vi "SVFA Power Spectrum Subset with Variable Resolution (1 Ch).vi"(0 "scaled signal [EU]":waveform(dbl)={"t0"=timestamp(0 s since 1904-01-01), "dt"=1e-05, "Y"=[]}, 2 "window":T2=1 items=["None"=0, "Hanning"=1, "Hamming"=2, "Blackman-Harris"=3, "Exact Blackman"=4, "Blackman"=5, "Flat Top"=6, "4 Term B-Harris "=7, "7 Term B-Harris"=8, "Low Sidelobe"=9, "Force"=64, "Exponential"=65, "Blackman Nuttall"=11, "Triangle"=30, "Bartlett-Hanning"=31, "Bohman"=32, "Parzen"=33, "Welch"=34, "Kaiser"=60, "Dolph-Chebyshev"=61, "Gaussian"=62], 3 "band specifications [Hz]":T1(array[cluster])=[{"start"=0.0, "stop"=500.0, "resolution"=3.6}, {"start"=500.0, "stop"=1600.0, "resolution"=6.25}, {"start"=1600.0, "stop"=3200.0, "resolution"=12.5}, {"start"=3200.0, "stop"=6400.0, "resolution"=25.0}, {"start"=6400.0, "stop"=12800.0, "resolution"=50.0}, {"start"=12800.0, "stop"=20000.0, "resolution"=100.0}], 4 "dB On (T)":bool=TRUE, 5 "error in (no error)":errorcluster) -> (14 "power spectrum [dB EU]":cluster{"frequencies":dbl[], "magnitudes":dbl[]} {"frequencies" format="%.2f"; "magnitudes" format="%.2p"}, 19 "error out":errorcluster)   [LabVIEW 2017]
uses:
  <vilib>/addons/_NISVFA/_Shared subVIs/Controls/svc_Window.ctl
  <vilib>/addons/_NISVFA/_Shared subVIs/Common/svc_Get Array Subset (Index).vi
  <vilib>/addons/_NISVFA/_Shared subVIs/Common/svc_Coerce Index and Length.vi
  <vilib>/addons/_NISVFA/_Shared subVIs/Common/svc_Conditional Merge Error.vi
  <vilib>/addons/_NISVFA/_Subset FFT/SVFA Power Spectrum Subset (1 Ch).vi
  <vilib>/measure/macond.llb/IIR Filter for 1 Chan.vi
  <vilib>/measure/NI_MAPro.lvlib
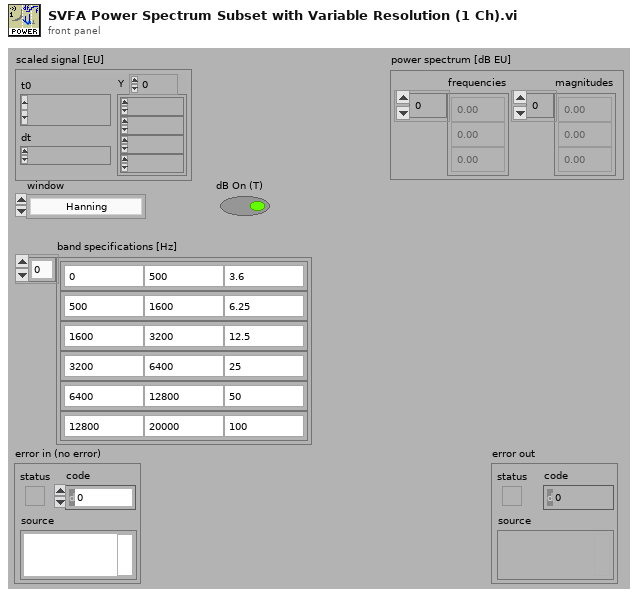
[diagram p1: front panel]
types:
  T1 = cluster{"start":dbl, "stop":dbl, "resolution":dbl}[]
  T2 = typedef "svc_Window.ctl" = u32
  T3 = cluster{"Topology":enum16{"Off", "Butterworth", "Chebyshev", "Inverse Chebyshev", "Elliptic", "Bessel"}, "Type":enum16{"Lowpass", "Highpass", "Bandpass", "Bandstop"}, "Order":i32, "Lower Fc":dbl, "Upper Fc":dbl, "PB Ripple":dbl, "SB Attenuation":dbl}
  T4 = cluster{"averaging mode":enum16{"No averaging", "Vector averaging", "RMS averaging", "Peak hold"}, "weighting mode":enum16{"Linear", "Exponential"}, "number of averages":u32, "linear mode":enum16{"One shot", "Auto restart"}}
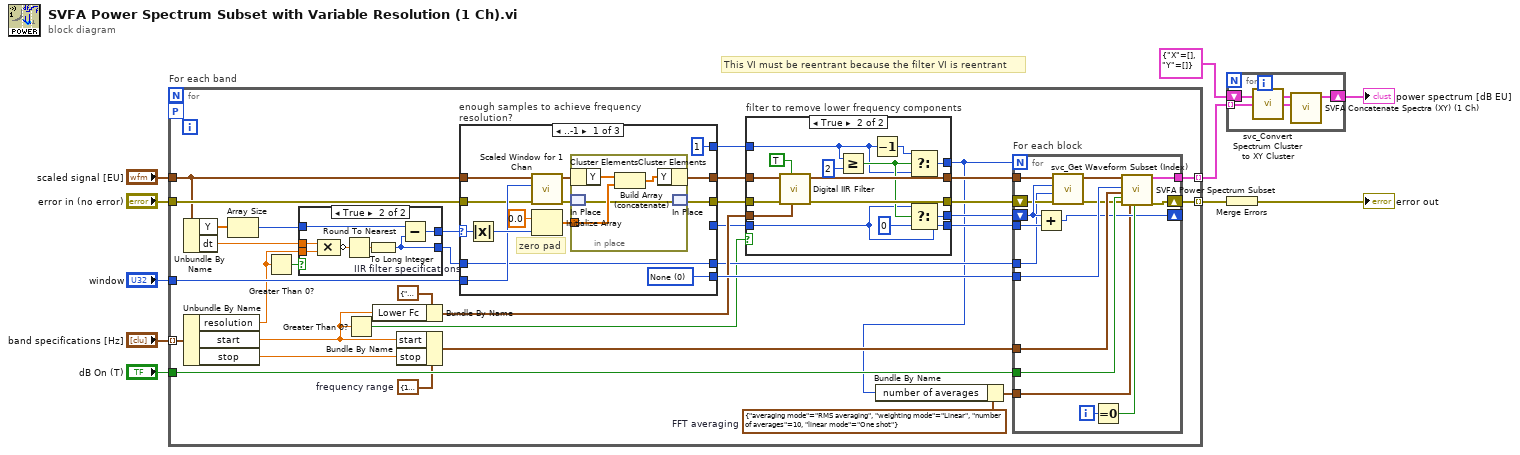
[diagram p0: block diagram]
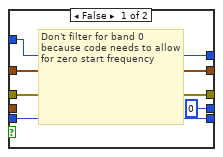
[diagram p2: hidden frame]
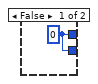
[diagram p3: hidden frame]
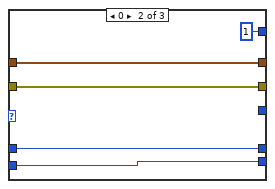
[diagram p4: hidden frame]
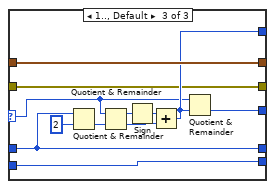
[diagram p5: hidden frame]
diagram:
  # "This VI must be reentrant because the filter VI is reentrant"
  n1 = for "For each band" {
    tunnel: "window" -> [w44]
    tunnel: "dB On (T)" -> [w39]
    tunnel: "band specifications [Hz]" -> [w25] mode=indexing
    tunnel: "scaled signal [EU]" -> [w14]
    tunnel: "error in (no error)" -> [w17]
    tunnel: [w38] -> w6 mode=indexing
    workers-P: _ -> [_]
    tunnel: [w15] -> w3 mode=indexing
    w22 = cluster{"start":dbl, "stop":dbl} {"start"=1000.0, "stop"=2000.0}  # frequency range
    w34 = T3 {"Topology"=enum."Chebyshev", "Type"=enum."Highpass", "Order"=6, "Lower Fc"=100.0, "Upper Fc"=200.0, "PB Ripple"=0.02, "SB Attenuation"=60.0}  # IIR filter specifications
    w36 = T4 {"averaging mode"=enum."RMS averaging", "weighting mode"=enum."Linear", "number of averages"=10, "linear mode"=enum."One shot"}  # FFT averaging
    n2 = Unbundle By Name(w14) -> ("Y"=w12:dbl[], "dt"=w11:dbl)
    n3 = Unbundle By Name(w25) -> ("resolution"=w24:dbl, "start"=w18:dbl, "stop"=w23:dbl)
    n4 = Array Size(array=w12) -> (size(s)=w13:i32)
    n5 = Greater Than 0?(x=w24) -> (x > 0?=w42:bool)
    n6 = case shown="True" w42 {
      tunnel: w11 -> [_ w87]
      tunnel: w24 -> [_ w86]
      tunnel: w13 -> [_ w85]
      tunnel: [w80 w82] -> w43
      tunnel: [w80 w81] -> w37
      frame False {
        w80 = 0
      }
      frame True {
        n7 = Compound Arithmetic op=MULTIPLY(w87, w86) -> (invert w84:dbl)
        n8 = Round To Nearest(number=w84) -> (nearest integer value=w83:dbl)
        n9 = To Long Integer(number=w83) -> (32bit integer=w81:i32)
        n10 = Subtract(x=w85, y=w81) -> (x-y=w82:i32)
      }
    }
    n11 = Greater Than 0?(x=w18) -> (x > 0?=w19:bool)
    n12 = Bundle By Name(cluster=w34, "Lower Fc"=w18) -> (w31:T3)
    n13 = Bundle By Name(cluster=w22, "start"=w18, "stop"=w23) -> (w40:cluster{"start":dbl, "stop":dbl})
    n14 = case "enough samples to achieve frequency resolution?" shown="..-1" w43 {
      selector: w43 -> [w101 _ w111]
      tunnel: w44 -> [w92 w109 w121]
      tunnel: w14 -> [w94 w110 w122]
      tunnel: [w98 w110 w122] -> w33
      tunnel: w37 -> [w91 w107 w113]
      tunnel: [w96 w109 w121] -> w41
      tunnel: [1 1 w115] -> w29
      tunnel: [_ _ w114] -> w28
      tunnel: [w91 w107 w113] -> w21
      tunnel: w17 -> [w90 w106 w112]
      tunnel: [w88 w106 w112] -> w16
      frame ..-1 {
        w96 = T2 0 items=["None"=0, "Hanning"=1, "Hamming"=2, "Blackman-Harris"=3, "Exact Blackman"=4, "Blackman"=5, "Flat Top"=6, "4 Term B-Harris "=7, "7 Term B-Harris"=8, "Low Sidelobe"=9, "Blackman Nuttall"=11, "Triangle"=30, "Bartlett-Hanning"=31, "Bohman"=32, "Parzen"=33, "Welch"=34, "Kaiser"=60, "Dolph-Chebyshev"=61, "Gaussian"=62] ("window")
        # "zero pad"
        n15 = Absolute Value(x=w101) -> (abs(x)=w97:i32)
        n16 = call <vilib>:"Scaled Window for 1 Chan.vi"("error in (no error)"=w90, "window"=w92, "signal in"=w94) -> ("error out"=w89:errorcluster, "signal out"=w93:waveform(dbl))  [unwired: 6 in, 1 out]
        n17 = Initialize Array(0.0 ("element"), w97) -> (w99:dbl[])
        n18 = in-place {
          in-place-border: w99 -> [w104]
          n19 = in-place-cluster #1(w93) -> ("Y"=w105:dbl[])
          n20 = in-place-match #2(w89) -> (w102:errorcluster)
          n21 = Build Array (concatenate)(w105, w104) -> (w103:dbl[])
          n22 = in-place-cluster #1("Y"=w103) -> (w98:waveform(dbl))
          n23 = in-place-match #2(w102) -> (w88:errorcluster)
        }
      }
      frame 0 {
      }
      frame 1.., Default {
        n24 = Quotient & Remainder(x=w113, y=2) -> (floor(x/y)=w119:i32)  [unwired: 1 out]
        n25 = Quotient & Remainder(x=w111, y=w119) -> (x-y*floor(x/y)=w118:i32, floor(x/y)=w116:i32)
        n26 = Sign(1:w118) -> (0:w117:i32)
        n27 = Add(x=w117, y=w116) -> (x+y=w115:i32)
        n28 = Quotient & Remainder(x=w111, y=w115) -> (floor(x/y)=w114:i32)  [unwired: 1 out]
      }
    }
    n29 = case "filter to remove lower frequency components" shown="True" w19 {
      tunnel: w33 -> [w48 w63]
      tunnel: w16 -> [w47 w62]
      tunnel: [w47 w61] -> w32
      tunnel: w31 -> [_ w60]
      tunnel: [w48 w59] -> w30
      tunnel: w29 -> [w49 w52]
      tunnel: [w49 w53] -> w20
      tunnel: w28 -> [w46 w51]
      tunnel: [w46 w51] -> w27
      tunnel: [0 ("f") w54] -> w26
      frame False {
        # "Don't filter for band 0 because code needs to allow for zero start frequency"
      }
      frame True {
        n30 = call-poly <vilib>:"Digital IIR Filter.vi"("IIR filter specifications"=w60, "reset filter"=TRUE, "error in (no error)"=w62, "signal in"=w63) -> ("error out"=w61:errorcluster, "signal out"=w59:waveform(dbl))  [unwired: 5 in, 1 out]
        n31 = Greater Or Equal?(x=w52, y=2) -> (x >= y?=w56:bool)
        n32 = Decrement(x=w52) -> (x-1=w57:i32)
        n33 = Select(t=w57, s=w56, f=w52) -> (s? t:f=w53:i32)
        n34 = Select(t=w51, s=w56, f=0) -> (s? t:f=w54:i32)
      }
    }
    n35 = Bundle By Name(cluster=w36, "number of averages"=w20) -> (w35:T4)
    n36 = for "For each block" {
      N: w20 -> [_]
      tunnel: w41 -> [w79]
      tunnel: [w78] -> w15
      tunnel: w40 -> [w75]
      tunnel: w39 -> [w74]
      shift-right: [w65] -> w38
      shift-left: w32 -> [w67]
      shift-right: [w70] -> _
      shift-left: w26 -> [w71]
      tunnel: w27 -> [w72]
      tunnel: w35 -> [w69]
      tunnel: w30 -> [w68]
      tunnel: w21 -> [w64]
      i -> [w77]
      n37 = Add(x=w71, y=w72) -> (x+y=w70:i32)
      n38 = call <vilib>:"svc_Get Waveform Subset (Index).vi"("error in (no error)"=w67, "length (-1 = all)"=w64, "start index (0)"=w71, "waveform in"=w68) -> ("error out"=w66:errorcluster, "waveform subset"=w73:waveform(dbl))  [unwired: 2 in, 4 out]
      n39 = Equal To 0?(x=w77) -> (x = 0?=w76:bool)
      n40 = call-poly <vilib>:"SVFA Power Spectrum Subset.vi"("scaled signal [EU]"=w73, "window"=w79, "frequency range"=w75, "dB On (T)"=w74, "error in (no error)"=w66, "averaging parameters"=w69, "restart averaging (F)"=w76) -> ("power spectrum [dB EU]"=w78:cluster{"f0":dbl, "df":dbl, "magnitude":dbl[]}, "error out"=w65:errorcluster)  [unwired: 7 in, 4 out]
    }
  }
  n41 = for {
    tunnel: w3 -> [w124] mode=indexing
    shift-right: [w125] -> w1
    shift-left: cluster{"X":dbl[], "Y":dbl[]} {"X"=[], "Y"=[]} ("XY cluster") -> [w126]
    n42 = call <vilib>:"svc_Convert Spectrum Cluster to XY Cluster.vi"("spectrum cluster"=w124) -> ("XY cluster"=w123:cluster{"X":dbl[], "Y":dbl[]})  [unwired: 4 in]
    n43 = call <vilib>:"SVFA Concatenate Spectra (XY) (1 Ch).vi"("spectrum (high frequency)"=w123, "spectrum (low frequency)"=w126) -> ("concatenated spectrum"=w125:cluster{"X":dbl[], "Y":dbl[]})  [unwired: 9 in]
  }
  "power spectrum [dB EU]" <- w1
  n44 = Merge Errors(w6) -> (→"error out":errorcluster)
